vi "Self Test.vi"(8 "error in":errorcluster, 10 "Board Image":T2, 11 "Resistor in":refnum<class "Resistor.lvclass">) -> (0 "error out":errorcluster, 2 "pass?":T1, 3 "Resistor out":refnum<class "Resistor.lvclass">)   [LabVIEW 2023, in "Resistor.lvclass"]
doc: "Check the image for this component's placement on the board."
uses:
  Resistor.lvclass
  c:/dev/_r/4/eng/lv-core/lvpostprocessingd/lv_mc_x86_64/dist_i386/examples/Object-Oriented Programming/Board Testing/Object Design/Component/Component.lvclass
  Common/Board Image.ctl
  Common/Pass Fail Boolean.ctl
  Component/Component.lvclass
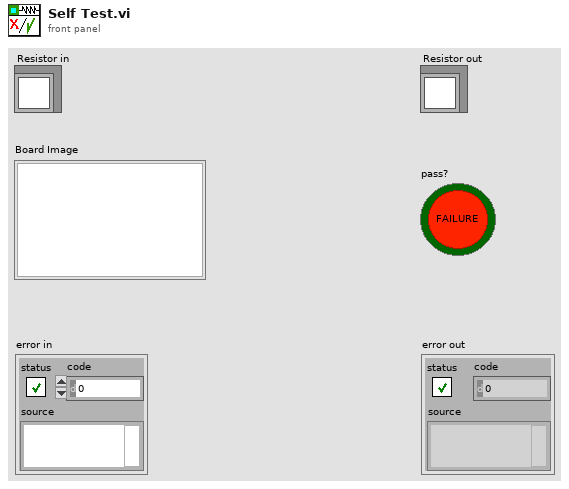
[diagram p1: front panel]
types:
  T1 = typedef "Pass Fail Boolean.ctl" = bool
  T2 = typedef "Board Image.ctl" = picture
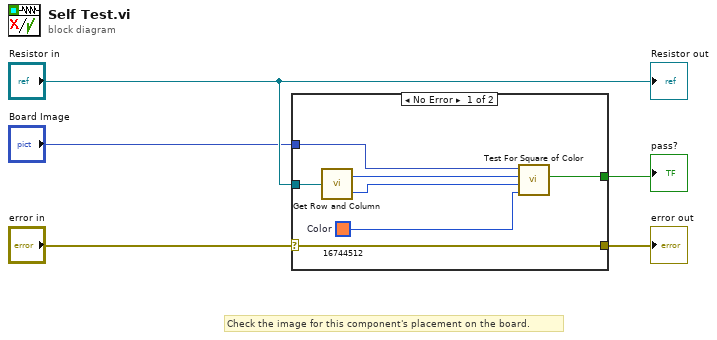
[diagram p0: block diagram]
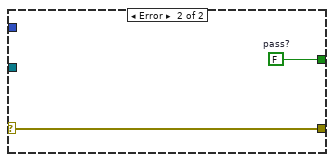
[diagram p2: hidden frame]
diagram:
  # "Check the image for this component's placement on the board."
  n1 = case shown="No Error" "error in" {
    selector: "error in" -> [w11 w14]
    tunnel: [w12 w13] -> w5
    tunnel: [w11 w14] -> w3
    tunnel: "Resistor in" -> [w9 _]
    tunnel: "Board Image" -> [w6 _]
    frame No Error {
      w10 = u32 16744512  # Color
      n2 = call "Get Row and Column.vi"("Component in"=w9) -> ("row"=w8:i16, "column"=w7:i16)
      n3 = call "Test For Square of Color.vi"("color"=w10, "column"=w7, "row"=w8, "board image"=w6) -> ("pass?"=w12:T1)  [unwired: 7 in]
    }
    frame Error {
      w13 = T1 FALSE  # pass?
    }
  }
  "error out" <- w3
  "pass?" <- w5
  "Resistor out" <- "Resistor in"
